vi "processor test.vi"() -> ()   [LabVIEW 2025]
uses:
  Classes/Processor/Processor.lvclass
panel:
  out "x = y?":bool
  out "Processor out 2":refnum<class "Processor.lvclass">
  out "Processor out":refnum<class "Processor.lvclass">
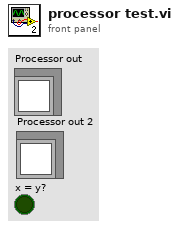
[diagram p1: front panel]
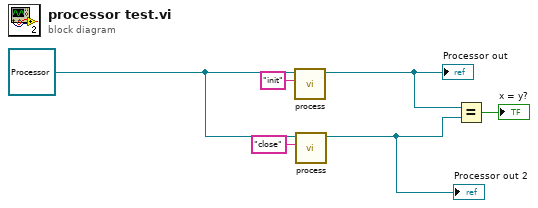
[diagram p0: block diagram]
diagram:
  w5 = refnum<class "Processor.lvclass"> refnum ("Processor.lvclass")
  n1 = call-dynamic "process.vi"("Process"="init", "Processor in"=w5) -> ("Processor out"=w3:refnum<class "Processor.lvclass">)  [unwired: 8 in, 1 out]
  "Processor out" <- w3
  n2 = call-dynamic "process.vi"("Process"="close", "Processor in"=w5) -> ("Processor out"=w2:refnum<class "Processor.lvclass">)  [unwired: 8 in, 1 out]
  "Processor out 2" <- w2
  n3 = Equal?(x=w3, y=w2) -> (x = y?=→"x = y?":bool)
